vi "DB_LeeVIF_HMI.vi"(8 "error in (no error)":errorcluster, 11 "ID_EQUIPO":i32=1) -> (0 "error out":errorcluster, 3 "Generador1":T1 {"I1" scale=0.0..1.0; "L1" scale=0.0..300.0; "Factor de Potencia" format="%#.1f"; "Potencia Total [kW]" format="%#.1f"; "Frecuencia [Hz]" format="%#.1f"; "I3" scale=0.0..1.0; "I2" scale=0.0..1.0; "L3" scale=0.0..300.0; "L2" scale=0.0..300.0})   [LabVIEW 2018]
uses:
  Controls/Cluster_HMI_VIFP - 2.ctl
  <vilib>/RAFA Solutions/Harmony UI Controls Kit/Numeric/Horizontal Progress Bar.ctl
  <vilib>/RAFA Solutions/Harmony UI Controls Kit/Numeric/Numeric Indicator.ctl
  <vilib>/addons/database/Connection.llb/DB Tools Open Connec (Path).vi
  <vilib>/addons/database/Connection.llb/Conn Execute.vi
  <vilib>/addons/database/Recordset.llb/Rec Fetch Recordset Data (R).vi
  <vilib>/addons/database/Recordset.llb/Rec Destroy - Connection.vi
  <vilib>/addons/database/_DB Variant To Data/Database Variant To Data.xnode
  <vilib>/addons/database/NI_Database_API.lvlib
  <vilib>/RAFA Solutions/Harmony UI Controls Kit/Flat UI Design.lvlib
panel:
  # "VOLTAJES [Vrms]"
  # "CORRIENTES [Arms]"
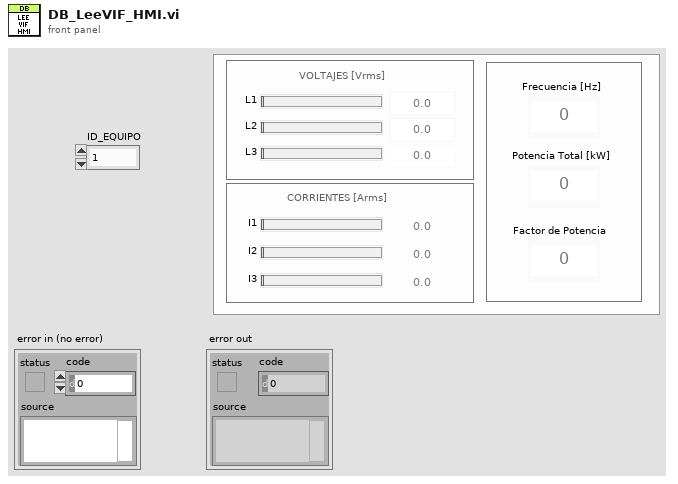
[diagram p1: front panel]
types:
  T1 = typedef "Cluster_HMI_VIFP - 2.ctl" = cluster{"L2":T2, "L3":T2, "I2":T2, "I3":T2, "Frecuencia [Hz]":T3, "Potencia Total [kW]":T3, "Factor de Potencia":T3, "L1":T2, "I1":T2}
  T2 = typedef "Flat UI Design.lvlib/Horizontal Progress Bar.ctl" = sgl
  T3 = typedef "Flat UI Design.lvlib/Numeric Indicator.ctl" = sgl
  T4 = typedef "NI_Database_API.lvlib/Conn ObjectReference.ctl" = refnum<k1>
  T5 = typedef "NI_Database_API.lvlib/Rec ObjectReference.ctl" = refnum<k1>
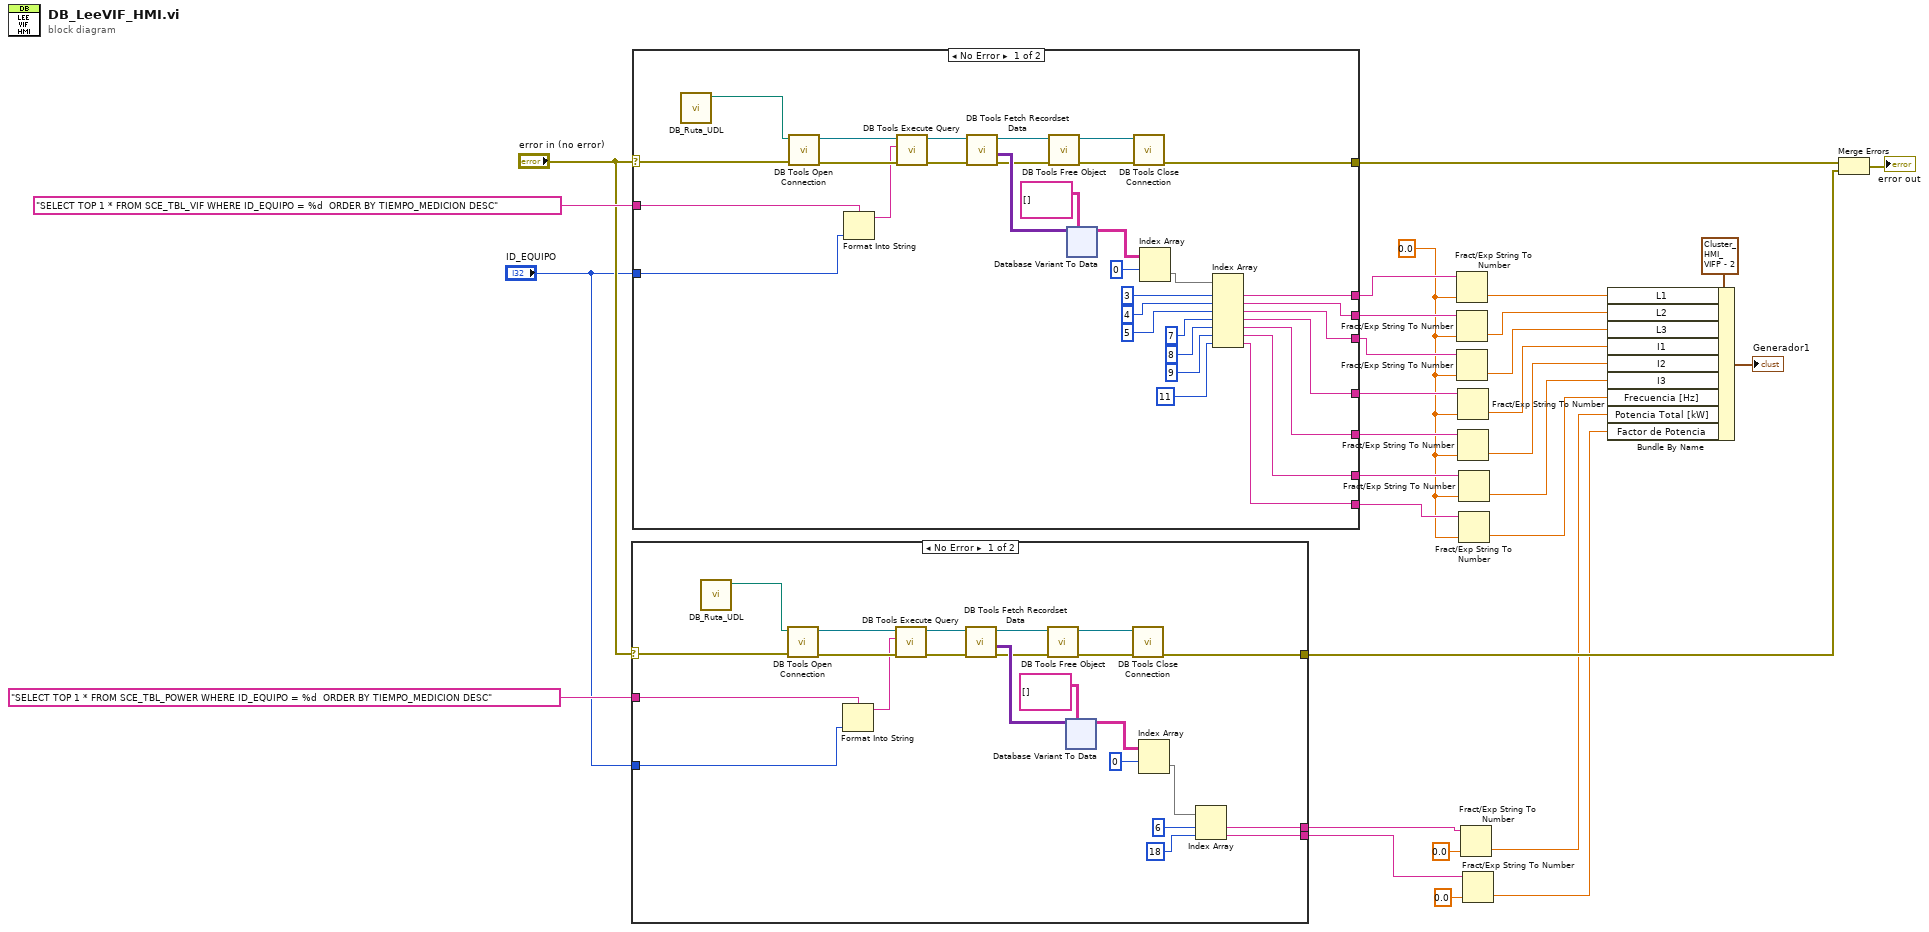
[diagram p0: block diagram]
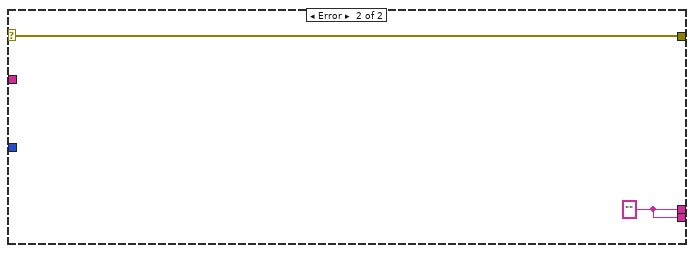
[diagram p2: hidden frame]
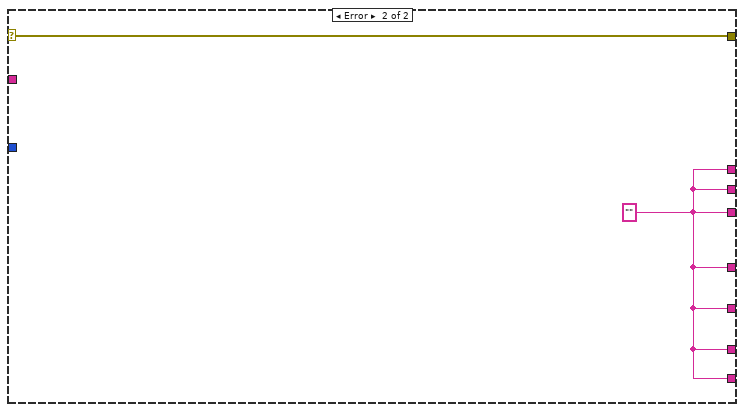
[diagram p3: hidden frame]
diagram:
  w1 = sgl 0.0
  n1 = case shown="No Error" "error in (no error)" {
    selector: "error in (no error)" -> [w48 w99]
    tunnel: [w50 w99] -> w25
    tunnel: "SELECT TOP 1 * FROM SCE_TBL_POWER WHERE ID_EQUIPO = %d  ORDER BY TIEMPO_MEDICION DESC" ("SQL") -> [w40 _]
    tunnel: [w36 w98] -> w6
    tunnel: "ID_EQUIPO" -> [w35 _]
    tunnel: [w33 w98] -> w5
    frame No Error {
      n2 = call "DB_Ruta_UDL.vi"() -> ("UDL ruta"=w32:path)  [unwired: 11 in]
      n3 = call-poly <vilib>:"DB Tools Open Connection.vi"("error in (no error)"=w48, "connection information"=w32) -> ("error out"=w53:errorcluster, "connection reference"=w51:T4)  [unwired: 6 in]
      n4 = Format Into String(format string=w40, w35) -> (resulting string=w39:string)  [unwired: 2 in, 1 out]
      n5 = call-poly <vilib>:"DB Tools Execute Query.vi"("error in (no error)"=w53, "SQL query"=w39, "connection reference"=w51) -> ("error out"=w49:errorcluster, "recordset reference"=w47:T5)  [unwired: 5 in]
      n6 = call-poly <vilib>:"DB Tools Fetch Recordset Data.vi"("error in (no error)"=w49, "recordset reference"=w47) -> ("error out"=w43:errorcluster, "recordset data"=w44:variant[][], "recordset reference out"=w46:T5)  [unwired: 3 in]
      n7 = call-poly <vilib>:"DB Tools Free Object.vi"("error in (no error)"=w43, "recordset reference"=w46) -> ("error out"=w52:errorcluster, "connection reference"=w31:T4)  [unwired: 8 in]
      n8 = xnode "Database Variant To Data"("database variant"=w44, "type"=string[][] []) -> ("data"=w42:string[][])  [unwired: 1 in, 1 out]
      n9 = call <vilib>:"DB Tools Close Connection.vi"("error in (no error)"=w52, "connection reference"=w31) -> ("error out"=w50:errorcluster)  [unwired: 5 in]
      n10 = Index Array(array=w42, index (row)=0 ("disabled index (col)")) -> (element=w38:string[])  [unwired: 1 in]
      n11 = Index Array(array=w38, index #1=6 ("index"), index #2=18 ("index")) -> (element #1=w36:string, element #2=w33:string)
    }
    frame Error {
      w98 = ""
    }
  }
  n12 = case shown="No Error" "error in (no error)" {
    selector: "error in (no error)" -> [w127 w178]
    tunnel: [w129 w178] -> w27
    tunnel: "SELECT TOP 1 * FROM SCE_TBL_VIF WHERE ID_EQUIPO = %d  ORDER BY TIEMPO_MEDICION DESC" ("SQL") -> [w119 _]
    tunnel: [w115 w177] -> w23
    tunnel: [w113 w177] -> w21
    tunnel: [w111 w177] -> w20
    tunnel: "ID_EQUIPO" -> [w110 _]
    tunnel: [w106 w177] -> w16
    tunnel: [w105 w177] -> w15
    tunnel: [w104 w177] -> w14
    tunnel: [w102 w177] -> w10
    frame No Error {
      n13 = call "DB_Ruta_UDL.vi"() -> ("UDL ruta"=w101:path)  [unwired: 11 in]
      n14 = call-poly <vilib>:"DB Tools Open Connection.vi"("error in (no error)"=w127, "connection information"=w101) -> ("error out"=w132:errorcluster, "connection reference"=w130:T4)  [unwired: 6 in]
      n15 = Format Into String(format string=w119, w110) -> (resulting string=w118:string)  [unwired: 2 in, 1 out]
      n16 = call-poly <vilib>:"DB Tools Execute Query.vi"("error in (no error)"=w132, "SQL query"=w118, "connection reference"=w130) -> ("error out"=w128:errorcluster, "recordset reference"=w126:T5)  [unwired: 5 in]
      n17 = call-poly <vilib>:"DB Tools Fetch Recordset Data.vi"("error in (no error)"=w128, "recordset reference"=w126) -> ("error out"=w122:errorcluster, "recordset data"=w123:variant[][], "recordset reference out"=w125:T5)  [unwired: 3 in]
      n18 = call-poly <vilib>:"DB Tools Free Object.vi"("error in (no error)"=w122, "recordset reference"=w125) -> ("error out"=w131:errorcluster, "connection reference"=w100:T4)  [unwired: 8 in]
      n19 = xnode "Database Variant To Data"("database variant"=w123, "type"=string[][] []) -> ("data"=w121:string[][])  [unwired: 1 in, 1 out]
      n20 = call <vilib>:"DB Tools Close Connection.vi"("error in (no error)"=w131, "connection reference"=w100) -> ("error out"=w129:errorcluster)  [unwired: 5 in]
      n21 = Index Array(array=w121, index (row)=0 ("disabled index (col)")) -> (element=w117:string[])  [unwired: 1 in]
      n22 = Index Array(array=w117, index #1=3 ("index"), index #2=4 ("index"), index #3=5 ("index"), index #4=7 ("index"), index #5=8 ("index"), index #6=9 ("index"), index #7=11 ("index")) -> (element #1=w115:string, element #2=w113:string, element #3=w111:string, element #4=w106:string, element #5=w105:string, element #6=w104:string, element #7=w102:string)
    }
    frame Error {
      w177 = ""
    }
  }
  n23 = Fract/Exp String To Number(string=w23, default (0 dbl)=w1) -> (number=w22:sgl)  [unwired: 2 in, 1 out]
  n24 = Fract/Exp String To Number(string=w21, default (0 dbl)=w1) -> (number=w19:sgl)  [unwired: 2 in, 1 out]
  n25 = Fract/Exp String To Number(string=w20, default (0 dbl)=w1) -> (number=w18:sgl)  [unwired: 2 in, 1 out]
  n26 = Fract/Exp String To Number(string=w16, default (0 dbl)=w1) -> (number=w13:sgl)  [unwired: 2 in, 1 out]
  n27 = Fract/Exp String To Number(string=w15, default (0 dbl)=w1) -> (number=w12:sgl)  [unwired: 2 in, 1 out]
  n28 = Fract/Exp String To Number(string=w14, default (0 dbl)=w1) -> (number=w11:sgl)  [unwired: 2 in, 1 out]
  n29 = Fract/Exp String To Number(string=w10, default (0 dbl)=w1) -> (number=w9:sgl)  [unwired: 2 in, 1 out]
  n30 = Fract/Exp String To Number(string=w6, default (0 dbl)=sgl 0.0) -> (number=w4:sgl)  [unwired: 2 in, 1 out]
  n31 = Fract/Exp String To Number(string=w5, default (0 dbl)=sgl 0.0) -> (number=w3:sgl)  [unwired: 2 in, 1 out]
  n32 = Bundle By Name(cluster=T1 {"L2"=0.0, "L3"=0.0, "I2"=0.0, "I3"=0.0, "Frecuencia [Hz]"=0.0, "Potencia Total [kW]"=0.0, "Factor de Potencia"=0.0, "L1"=0.0, "I1"=0.0} ("Generador1"), "L1"=w22, "L2"=w19, "L3"=w18, "I1"=w13, "I2"=w12, "I3"=w11, "Frecuencia [Hz]"=w9, "Potencia Total [kW]"=w4, "Factor de Potencia"=w3) -> (→"Generador1":T1)
  n33 = Merge Errors(w27, w25) -> (→"error out":errorcluster)
